vi "Write AI_index.vi"(9 "Reg":string, 10 "EnumsAI":string[](array[string]), 11 "bronkhorst_reg in":refnum<class "bronkhorst_reg_2.lvclass">) -> (2 "Find":bool, 3 "bronkhorst_reg out":refnum<class "bronkhorst_reg_2.lvclass">)   [LabVIEW 2019, in "control.lvlib" / "bronkhorst_reg_2.lvclass"]
uses:
  bronkhorst_reg_2.lvclass
  bronkhorst_reg_2.lvclass/bronkhorst_reg_2.ctl
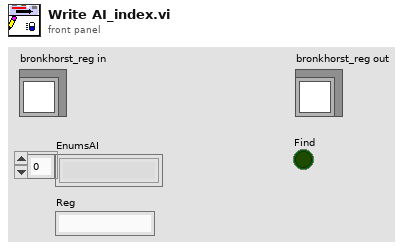
[diagram p1: front panel]
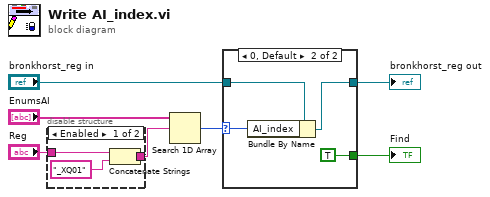
[diagram p0: block diagram]
diagram:
  n1 = disable-structure shown="Enabled" {
    disable-tunnel: "Reg" -> [w9 w11]
    disable-tunnel: [w8 w11] -> w1
    frame Enabled {
      n2 = Concatenate Strings(w9, "_XQ01" ("string")) -> (w8:string)
    }
    frame Disabled {
    }
  }
  n3 = Search 1D Array(1D array="EnumsAI", element=w1) -> (index of element=w4:i32)  [unwired: 1 in]
  n4 = case shown="0, Default" w4 {
    selector: w4 -> [_ w14]
    tunnel: "bronkhorst_reg in" -> [w12 w16]
    tunnel: [w12 w15] -> w6
    tunnel: [_ TRUE] -> w3
    frame -1 {
    }
    frame 0, Default {
      n5 = Bundle By Name(cluster=w16, "AI_index"=w14) -> (w15:refnum<class "bronkhorst_reg_2.lvclass">)
    }
  }
  "bronkhorst_reg out" <- w6
  "Find" <- w3
